vi "DeactivateAnalogVelocitySettingValue.vi"(4 "error in (no error)":errorcluster, 6 "analogInputNumber":u16, 7 "axis in":cluster{"keyHandle":u32, "nodeId":u16}={"keyHandle"=0, "nodeId"=1}) -> (0 "error out":errorcluster, 3 "axis out":cluster{"keyHandle":u32, "nodeId":u16}={"keyHandle"=0, "nodeId"=1})   [LabVIEW 2017, in "maxonEPOS.lvlib"]
doc: "<B>DeactivateAnalogVelocitySettingValue</B> disables the selected analog input for analog velocity setpoint."
uses:
  Examples/maxonEPOS.lvlib
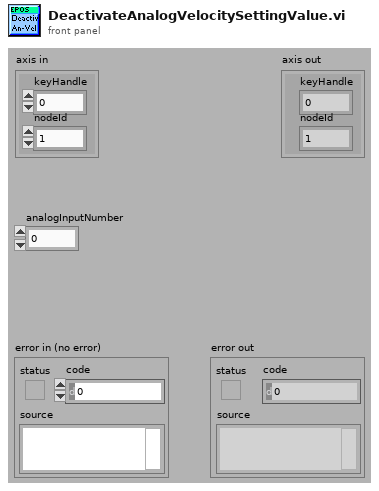
[diagram p1: front panel]
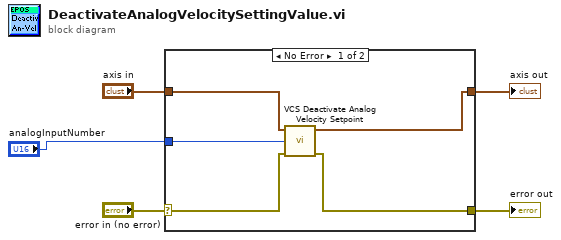
[diagram p0: block diagram]
diagram:
  n1 = case shown="No Error" "error in (no error)" {
    selector: "error in (no error)" -> [w7 w12]
    tunnel: [w10 w12] -> w4
    tunnel: [w9 w11] -> w3
    tunnel: "axis in" -> [w8 w11]
    tunnel: "analogInputNumber" -> [w6 _]
    frame No Error {
      n2 = call "VCS Deactivate Analog Velocity Setpoint.vi"("error in (no error)"=w7, "analogInputNumber"=w6, "axis in"=w8) -> ("error out"=w10:errorcluster, "axis out"=w9:cluster{"keyHandle":u32, "nodeId":u16})  [unwired: 7 in]
    }
    frame Error {
    }
  }
  "error out" <- w4
  "axis out" <- w3
